vi "Camera_info.vi"(0 "设备索引":i32[](array[numeric]), 5 "设备列表":u16(ring) items=["设备1_22592_3034"], 7 "DevCfgGet":cluster{"pid":u32, "vid":u32, "ser_num":u64}[](array[cluster]), 9 "分辨率数量上限":i32=15, 11 "error in":errorcluster) -> (4 "获取设备信息返回值":i32, 6 "camera_stream_info[]":T1(array[cluster]), 8 "分辨率索引":i32[](array[numeric]), 10 "分辨率":u16(ring) items=["256*192", "256*384", "256*192", "256*384"], 15 "error out":errorcluster)   [LabVIEW 2016]
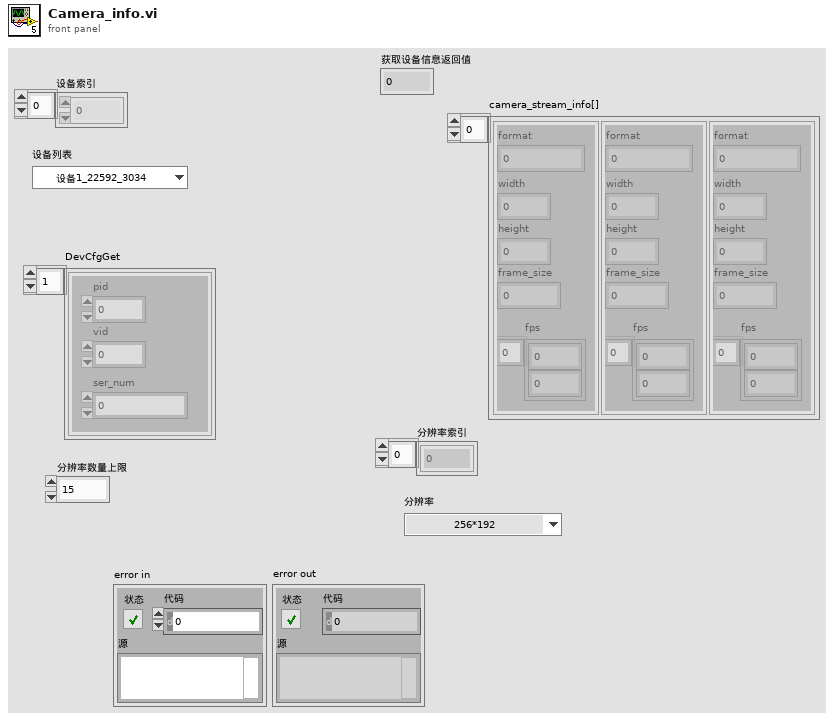
[diagram p1: front panel]
types:
  T1 = cluster{"format":u64, "width":u32, "height":u32, "frame_size":u32, "fps":u32[]}[]
  T2 = cluster{"format":u64, "width":u32, "height":u32, "frame_size":u32, "fps":u32[]}
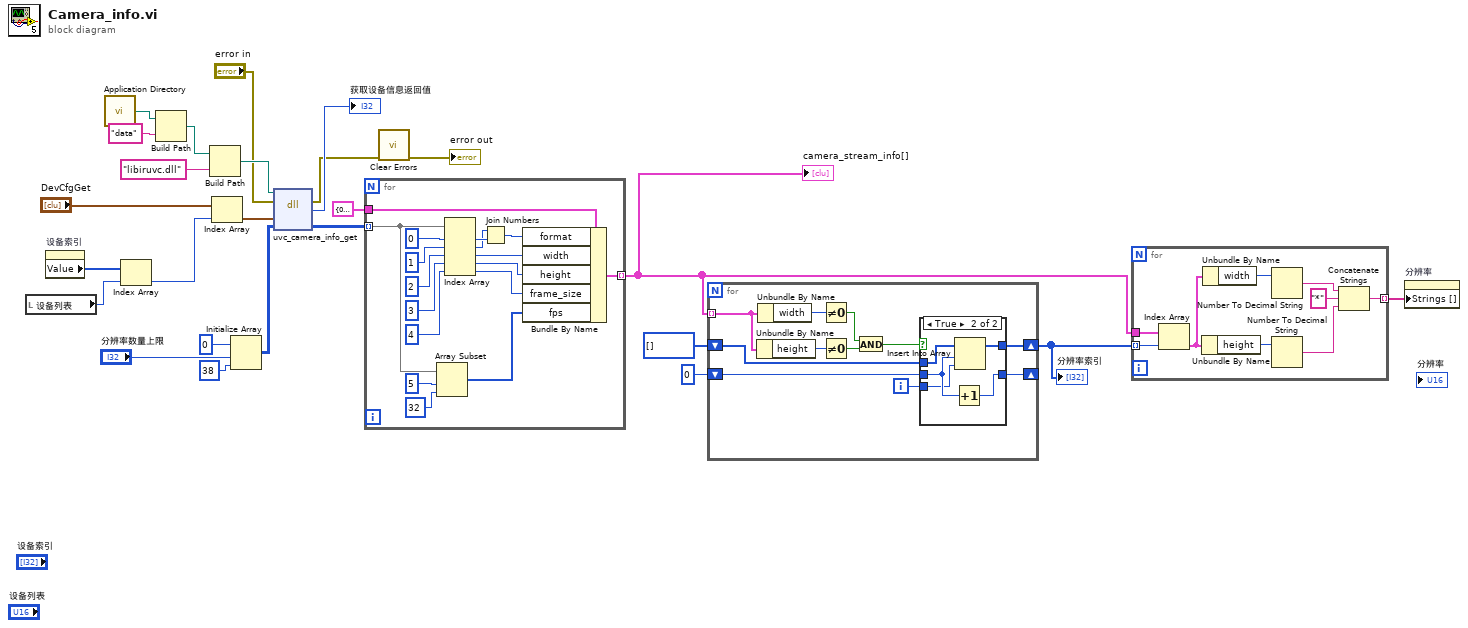
[diagram p0: block diagram]
diagram:
  n1 = local read "设备列表"() -> (w14:u16)
  n2 = property on="设备索引" class="Arr (strict)"() -> ("Value"=w15:i32[])  [unwired: 2 in, 2 out]
  n3 = call <vilib>:"Application Directory.vi"() -> ("Application Directory"=w22:path)
  n4 = Index Array(array=w15, index=w14) -> (element=w13:i32)
  n5 = Build Path(base path=w22, name or relative path="data") -> (appended path=w21:path)
  n6 = Build Path(base path=w21, name or relative path="libiruvc.dll") -> (appended path=w24:path)
  n7 = Index Array(array="DevCfgGet", index=w13) -> (element=w25:cluster{"pid":u32, "vid":u32, "ser_num":u64})
  n8 = Initialize Array(u32 0, "分辨率数量上限", 38) -> (w17:u32[][])
  n9 = dll-call lib="D:/libiruvc_0.3.3/windows/x64/dll/libiruvc.dll" fn="uvc_camera_info_get"(path in=w24, error in="error in", "dev_cfg"=w25, "camera_stream_info[]"=w17) -> (error out=w2:errorcluster, "return type"=→"获取设备信息返回值":i32, "camera_stream_info[]"=w16:u32[][])  [unwired: 2 in, 1 out]
  n10 = for {
    tunnel: w16 -> [w35] mode=indexing
    tunnel: T2 {"format"=0, "width"=0, "height"=0, "frame_size"=0, "fps"=[]} ("CameraStreamInfo") -> [w34]
    tunnel: [w31] -> w7 mode=indexing
    n11 = Array Subset(array=w35, index=5, length=32) -> (w33:u32[])
    n12 = Index Array(array=w35, index #1=0, index #2=1, index #3=2, index #4=3, index #5=4) -> (element #1=w30:u32, element #2=w29:u32, element #3=w27:u32, element #4=w26:u32, element #5=w32:u32)
    n13 = Join Numbers(hi=w29, lo=w30) -> ((hi.lo)=w28:u64)
    n14 = Bundle By Name(cluster=w34, "format"=w28, "width"=w27, "height"=w26, "frame_size"=w32, "fps"=w33) -> (w31:T2)
  }
  "camera_stream_info[]" <- w7
  n15 = call <vilib>:"Clear Errors.vi"("error in (no error)"=w2) -> ("error out"=→"error out":errorcluster)  [unwired: 5 in, 1 out]
  n16 = for {
    tunnel: w7 -> [w53] mode=indexing
    shift-right: [w45] -> w10
    shift-left: i32[] [] -> [w47]
    shift-right: [w44] -> _
    shift-left: 0 -> [w46]
    i -> [w43]
    n17 = Unbundle By Name(w53) -> ("height"=w51:u32)
    n18 = Unbundle By Name(w53) -> ("width"=w52:u32)
    n19 = Not Equal To 0?(x=w52) -> (x != 0?=w50:bool)
    n20 = Not Equal To 0?(x=w51) -> (x != 0?=w49:bool)
    n21 = And(x=w50, y=w49) -> (x .and. y?=w48:bool)
    n22 = case shown="True" w48 {
      tunnel: w47 -> [w55 w60]
      tunnel: w46 -> [w54 w58]
      tunnel: [w55 w59] -> w45
      tunnel: [w54 w57] -> w44
      tunnel: w43 -> [_ w56]
      frame False {
      }
      frame True {
        n23 = Increment(x=w58) -> (x+1=w57:i32)
        n24 = Insert Into Array(array=w60, index=w58, new element=w56) -> (w59:i32[])
      }
    }
  }
  "分辨率索引" <- w10
  n25 = for {
    tunnel: w10 -> [w63] mode=indexing
    tunnel: w7 -> [w62]
    tunnel: [w64] -> w9 mode=indexing
    n26 = Index Array(array=w62, index=w63) -> (element=w61:T2)
    n27 = Unbundle By Name(w61) -> ("height"=w69:u32)
    n28 = Unbundle By Name(w61) -> ("width"=w68:u32)
    n29 = Number To Decimal String(number=w68) -> (decimal integer string=w65:string)  [unwired: 1 in]
    n30 = Number To Decimal String(number=w69) -> (decimal integer string=w67:string)  [unwired: 1 in]
    n31 = Concatenate Strings(w65, "*", w67) -> (w64:string)
  }
  n32 = property on="分辨率" class="Ring (strict)"("Strings []"=w9) -> ()  [unwired: 2 in, 2 out]
